vi "get update file.vi"(8 "error in (no error)":errorcluster, 11 "远端地址":string="/updatefiles/OneStation/V4/一体化微型水质监测站.zip") -> (0 "error out":errorcluster)   [LabVIEW 2016, in "数据传输系统-02.lvlib" / "update.lvlib"]
uses:
  update.lvlib
  http client class/http client.lvclass
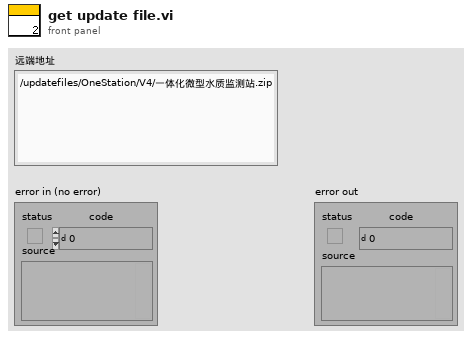
[diagram p1: front panel]
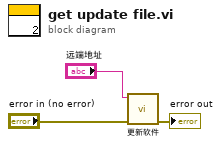
[diagram p0: block diagram]
diagram:
  n1 = call "更新软件.vi"("error in (no error)"="error in (no error)", "远端地址"="远端地址") -> ("error out"=→"error out":errorcluster)  [unwired: 9 in]
